vi "L3.vi"() -> ()   [LabVIEW 2014]
panel:
  in  "stop":bool
  out "f(x)":i64
  in  "X":i64
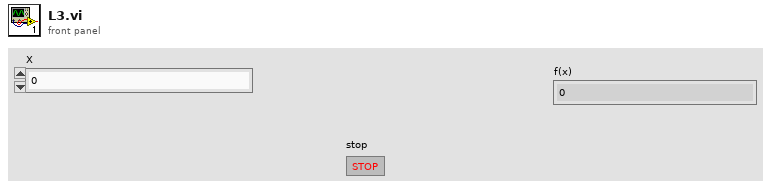
[diagram p1: front panel]
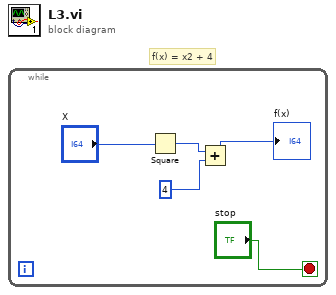
[diagram p0: block diagram]
diagram:
  # "f(x) = x2 + 4"
  n1 = while {
    stop <- "stop" stop-if-true
    n2 = Square(x="X") -> (x^2=w4:i64)
    n3 = Add(x=w4, y=4) -> (x+y=→"f(x)":i64)
  }
